vi "Array-Delete String and Parse Fields.vi"(0 "Array in":string[](array[string]), 9 "Separator":string=":") -> (4 "Array out":string[](array[string]), 8 "Field 1":string, 13 "Field 4":string, 14 "Field 3":string, 15 "Field 2":string)   [LabVIEW 2020]
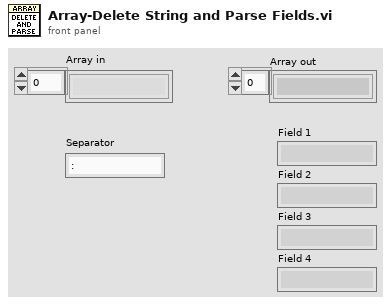
[diagram p1: front panel]
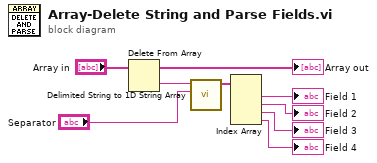
[diagram p0: block diagram]
diagram:
  n1 = Delete From Array(array="Array in") -> (deleted portion=w7:string, array with subset deleted=→"Array out":string[])  [unwired: 2 in]
  n2 = call <vilib>:"Delimited String to 1D String Array.vi"("delimiter"="Separator", "delimited string"=w7) -> ("string array"=w5:string[])  [unwired: 9 in]
  n3 = Index Array(array=w5) -> (element #1=→"Field 1":string, element #2=→"Field 2":string, element #3=→"Field 3":string, element #4=→"Field 4":string)  [unwired: 4 in]
